vi "Agilent 34420 Read Single Temperature.vi"() -> ()   [LabVIEW 2021]
doc: "This example shows how to configure a temperature measurement and take a reading."
uses:
  <instrlib>/Agilent 34420/Public/Configure/Configure Temperature (Thermistor).vi
  <instrlib>/Agilent 34420/Public/Data/Read (Single Point).vi
  <instrlib>/Agilent 34420/Agilent 34420.lvlib
panel:
  in  "Units (0: Celsius)":u16(ring) items=["Celsius", "Fahrenheit", "Kelvin"]
  out "Measurement":dbl
  in  "Serial Configuration":T1={"Baud Rate"=9600, "Parity"=0, "Data Bits"=8} {"Data Bits" items=["7"=7, "8"=8]; "Parity" items=["None", "Odd", "Even", "Mark", "Space"]; "Baud Rate" items=["300"=300, "600"=600, "1200"=1200, "2400"=2400, "4800"=4800, "9600"=9600]}
  in  "Auto Range (T: Enable)":bool=TRUE
  in  "Manual Range (1.0)":dbl=1.0
  in  "VISA resource name":refnum<visa-resource-name>
  # "(c) 2008-2015 National Instruments Corp.  ALL RIGHTS RESERVED."
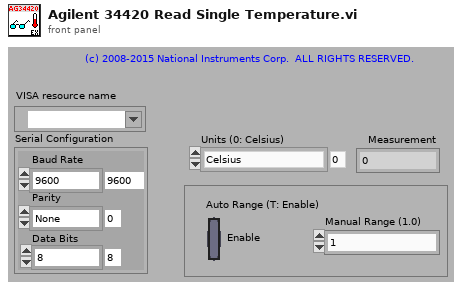
[diagram p1: front panel]
types:
  T1 = cluster{"Baud Rate":u32, "Parity":u16, "Data Bits":u16}
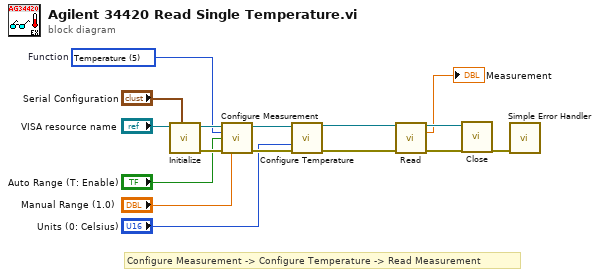
[diagram p0: block diagram]
diagram:
  w6 = u16 5 items=["DC Volts", "DC Voltage Ratio", "DC Voltage Difference", "2 Wire Resistance", "4 Wire Resistance", "Temperature"]  # Function
  # "Configure Measurement -> Configure Temperature -> Read Measurement"
  n1 = call <instrlib>:"Initialize.vi"("Serial Configuration"="Serial Configuration", "VISA resource name"="VISA resource name") -> ("error out"=w13:errorcluster, "VISA resource name out"=w14:refnum<visa-resource-name>)  [unwired: 8 in]
  n2 = call <instrlib>:"Configure Measurement.vi"("VISA resource name"=w14, "Function (0: DC Volts)"=w6, "Auto Range (T:Enable)"="Auto Range (T: Enable)", "error in (no error)"=w13, "Manual Range (0.001)"="Manual Range (1.0)") -> ("VISA resource name out"=w4:refnum<visa-resource-name>, "error out"=w5:errorcluster)  [unwired: 9 in]
  n3 = call-poly <instrlib>:"Configure Temperature.vi"("VISA resource name"=w4, "Units (0: Celsius)"="Units (0: Celsius)", "error in (no error)"=w5) -> ("VISA resource name out"=w2:refnum<visa-resource-name>, "error out"=w3:errorcluster)  [unwired: 11 in]
  n4 = call-poly <instrlib>:"Read.vi"("VISA resource name"=w2, "error in (no error)"=w3) -> ("VISA resource name out"=w10:refnum<visa-resource-name>, "Measurement"=→"Measurement":dbl, "error out"=w11:errorcluster)  [unwired: 11 in]
  n5 = call <instrlib>:"Close.vi"("error in (no error)"=w11, "VISA resource name"=w10) -> ("error out"=w16:errorcluster)  [unwired: 9 in]
  n6 = call <vilib>:"Simple Error Handler.vi"("error in (no error)"=w16) -> ()  [unwired: 4 in, 5 out]
